vi "Pre Enqueue Action.vi"(8 "error in (no error)":errorcluster, 10 "Message Array in":refnum<class "Message.lvclass">[](array[class]), 11 "Msg in":refnum<class "Loop Msg.lvclass">) -> (0 "error out":errorcluster, 2 "Message Array out":refnum<class "Message.lvclass">[](array[class]))   [LabVIEW 2020, in "Sequencer.lvlib" / "Loop Msg.lvclass"]
doc: "Action performed on the message array prior to the enqueue on the Sequencer Core.\n\nThis implementation re-enqueues the Loop Msg at the end of the message array creating never ending loop. An external interrupt is required to end the looping."
uses:
  Loop Msg.lvclass
  PPL/HDH.Actor Framework.Core.Actor.lvlibp/1abvi3w/vi.lib/ActorFramework/Message/Message.lvclass
  C:/Current projects/WS/PPL/HDH.Actor Framework.Core.Actor.lvlibp/1abvi3w/vi.lib/ActorFramework/Message/Message.lvclass
  Loop Msg.lvclass/Loop Msg.ctl
  PPL/HDH.Actor Framework.Core.Msg.lvlibp/Flex Msg/Flex Msg.lvclass
  PPL/HDH.Actor Framework.Core.Msg.lvlibp/Flex Msg/Data Access Handlers/Set Controls/Set Controls.lvclass
  C:/Current projects/WS/PPL/HDH.Actor Framework.Core.Msg.lvlibp/Flex Msg/Data Access Handlers/Data Access Handler/Data Access Handler.lvclass
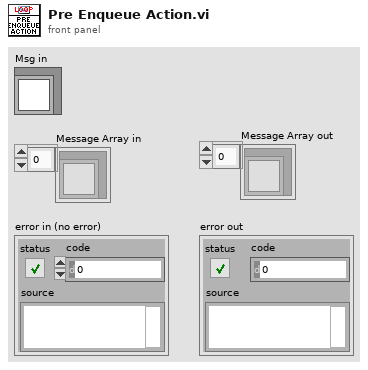
[diagram p1: front panel]
types:
  T1 = typedef "Sequencer.lvlib/Ctl_FlexDataElements.ctl" = cluster{"Flex Data":T2[]}
  T2 = typedef "Sequencer.lvlib/Ctl_FlexDataElement.ctl" = cluster{"Control Index":i32, "Data Values":variant[]}
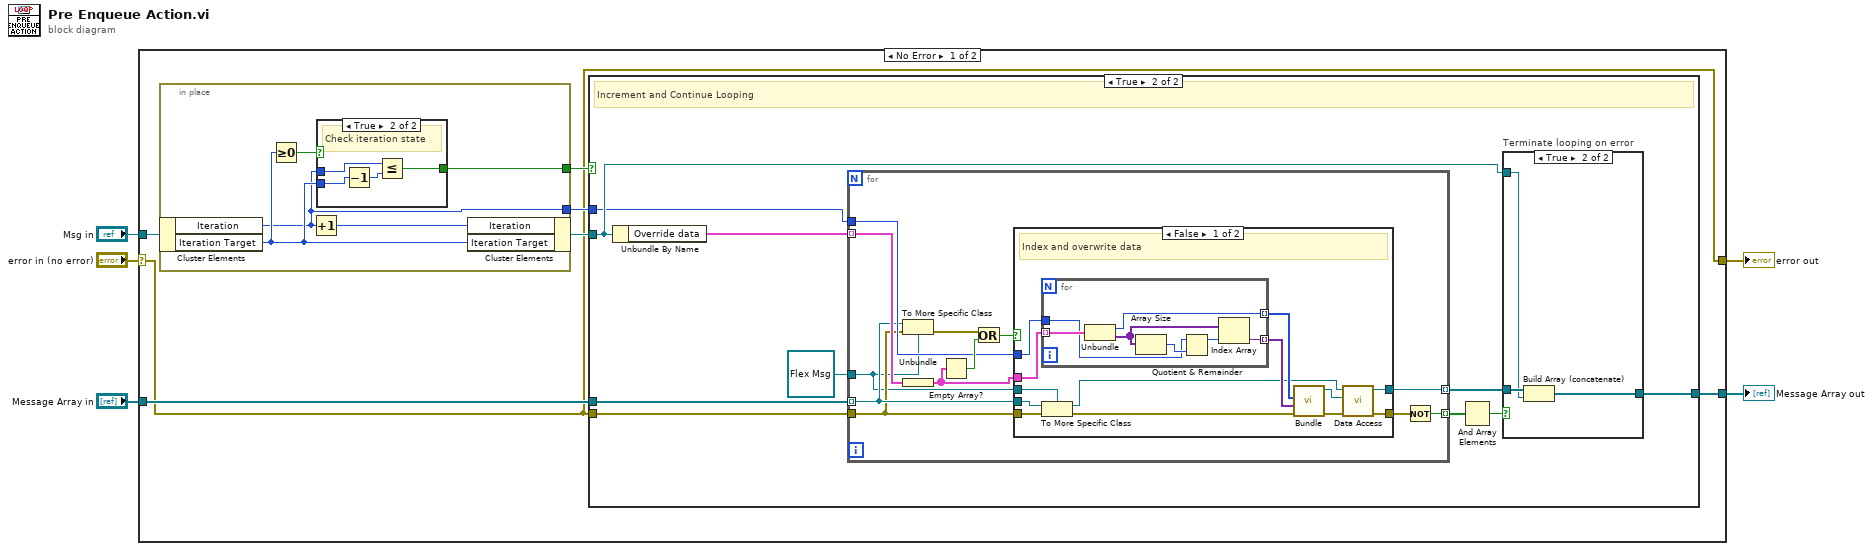
[diagram p0: block diagram]
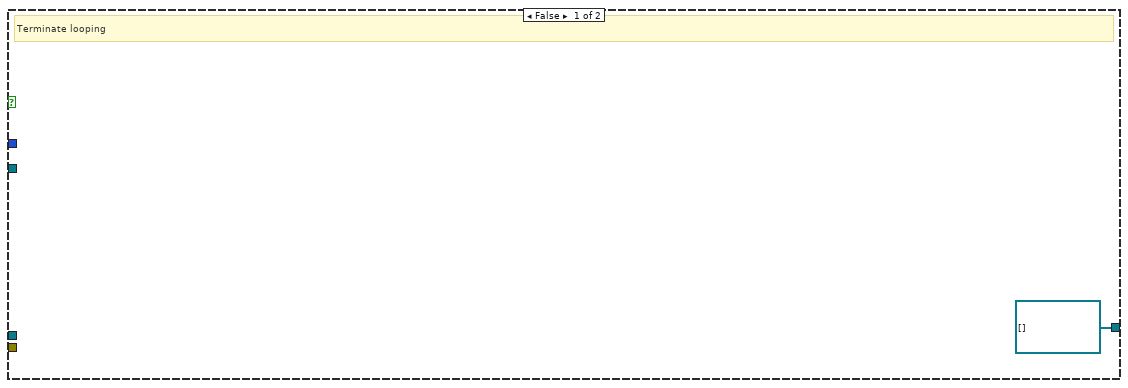
[diagram p2: hidden frame]
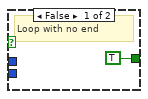
[diagram p5: hidden frame]
diagram:
  n1 = case shown="No Error" "error in (no error)" {
    selector: "error in (no error)" -> [w6 w71]
    tunnel: [w6 w71] -> w2
    tunnel: "Msg in" -> [w12 _]
    tunnel: "Message Array in" -> [w9 _]
    tunnel: [w10 _] -> w1
    frame No Error {
      n2 = in-place {
        in-place-border: [w63] -> w11
        in-place-border: [w61] -> w7
        n3 = in-place-cluster #1(w12) -> ("Iteration"=w61:i32, "Iteration Target"=w62:i32)
        n4 = Greater Or Equal To 0?(x=w62) -> (x >= 0?=w64:bool)
        n5 = Increment(x=w61) -> (x+1=w65:i32)
        n6 = case shown="True" w64 {
          tunnel: w61 -> [_ w70]
          tunnel: w62 -> [_ w69]
          tunnel: [TRUE w68] -> w63
          frame False {
            # "Loop with no end"
          }
          frame True {
            # "Check iteration state"
            n7 = Decrement(x=w69) -> (x-1=w67:i32)
            n8 = Less Or Equal?(x=w70, y=w67) -> (x <= y?=w68:bool)
          }
        }
        n9 = in-place-cluster #1("Iteration"=w65, "Iteration Target"=w62) -> (w8:refnum<class "Loop Msg.lvclass">)
      }
      n10 = case shown="True" w11 {
        tunnel: [refnum<class "Message.lvclass">[] [] ("Message Array out") w20] -> w10
        tunnel: w9 -> [_ w23]
        tunnel: w8 -> [_ w21]
        tunnel: w7 -> [_ w18]
        tunnel: w6 -> [_ w17]
        frame False {
          # "Terminate looping"
        }
        frame True {
          # "Increment and Continue Looping"
          n11 = Unbundle By Name(w21) -> ("Override data"=w19:T1[])
          n12 = for {
            tunnel: w19 -> [w38] mode=indexing
            tunnel: w23 -> [w33] mode=indexing
            tunnel: [w36] -> w22 mode=indexing
            tunnel: w18 -> [w34]
            tunnel: w17 -> [w30]
            tunnel: refnum<class "Flex Msg.lvclass"> refnum ("HDH.Actor Framework.Core.Msg.lvlibp:Flex Msg.lvclass") -> [w29]
            tunnel: [w27] -> w15 mode=indexing
            n13 = To More Specific Class(target class=w29, reference=w33, error in=w30) -> (error out=w31:errorcluster)  [unwired: 1 out]
            n14 = Unbundle(w38) -> ("Flex Data"=w35:T2[])
            n15 = Empty Array?(array=w35) -> (empty?=w37:bool)
            n16 = Or(x=w31, y=w37) -> (x .or. y?=w32:bool)
            n17 = case shown="False" w32 {
              tunnel: [w40 w60] -> w36
              tunnel: w33 -> [w46 w60]
              tunnel: w35 -> [w51 _]
              tunnel: w34 -> [w50 _]
              tunnel: w30 -> [w44 w59]
              tunnel: w29 -> [w45 _]
              tunnel: [w39 w59] -> w28
              frame False {
                # "Index and overwrite data"
                n18 = for {
                  tunnel: w51 -> [w58] mode=indexing
                  tunnel: [w57] -> w49 mode=indexing
                  tunnel: w50 -> [w55]
                  tunnel: [w52] -> w48 mode=indexing
                  n19 = Unbundle(w58) -> ("Control Index"=w57:i32, "Data Values"=w53:variant[])
                  n20 = Array Size(array=w53) -> (size(s)=w56:i32)
                  n21 = Quotient & Remainder(x=w55, y=w56) -> (x-y*floor(x/y)=w54:i32)  [unwired: 1 out]
                  n22 = Index Array(array=w53, index=w54) -> (element=w52:variant)
                }
                n23 = To More Specific Class(target class=w45, reference=w46, error in=w44) -> (specific class reference=w43:refnum<class "Flex Msg.lvclass">, error out=w42:errorcluster)
                n24 = call "Bundle.vi"("error in (no error)"=w42, "Data Values"=w48, "Control Indices"=w49) -> ("error out"=w41:errorcluster, "Set Controls out"=w47:refnum<class "Set Controls.lvclass">)  [unwired: 7 in]
                n25 = call-dynamic "Data Access.vi"("error in (no error)"=w41, "Data Access Handler"=w47, "Flex Msg in"=w43) -> ("error out"=w39:errorcluster, "Flex Msg out"=w40:refnum<class "Flex Msg.lvclass">)  [unwired: 7 in]
              }
              frame True {
                # "Nothing to overwrite"
              }
            }
            n26 = Not(x=w28) -> (.not. x?=w27:bool)
          }
          n27 = And Array Elements(Boolean array=w15) -> (logical AND=w14:bool)
          n28 = case "Terminate looping on error" shown="True" w14 {
            tunnel: w22 -> [_ w26]
            tunnel: w21 -> [_ w25]
            tunnel: [_ w24] -> w20
            frame False {
            }
            frame True {
              n29 = Build Array (concatenate)(w26, w25) -> (w24:refnum<class "Message.lvclass">[])
            }
          }
        }
      }
    }
    frame Error {
    }
  }
  "Message Array out" <- w1
  "error out" <- w2
